vi "GetCurrentVideoDriver.vi"(8 "No Error":errorcluster) -> (0 "Error Out":errorcluster, 3 "Video Driver":string)   [LabVIEW 2026, in "SDL3.lvlib" / "Video.lvlib"]
doc: "<B>Summary</B>\nGet the name of the currently initialized video driver.\n\n<B>Remarks</B>\nThe names of drivers are all simple, low-ASCII identifiers, like \"cocoa\", \"x11\" or \"windows\". These never have Unicode characters, and are not meant to be proper names."
uses:
  Video.lvlib
  Lib/SDL3.dll
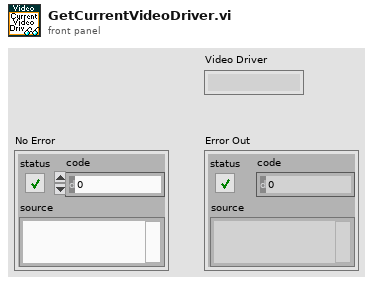
[diagram p1: front panel]
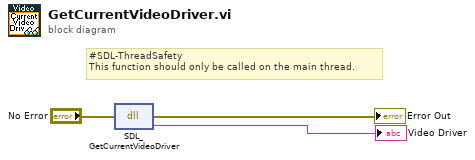
[diagram p0: block diagram]
diagram:
  # "#SDL-ThreadSafety\nThis function should only be called on the main thread."
  n1 = dll-call lib="C:/Users/saukko/Dev/LV-SDL3/Sources/SDL3/Lib/SDL3.*" fn="SDL_GetCurrentVideoDriver"(error in="No Error") -> (error out=→"Error Out":errorcluster, "return type"=→"Video Driver":string)  [unwired: 2 in, 1 out]
